vi "sub_panel_queue.vi"() -> ()   [LabVIEW 2024]
panel:
  out "Boolean":bool
  in  "knob":dbl(knob) scale=0.0..10.0
  out "numeric_test":dbl
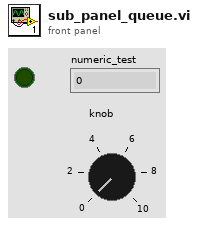
[diagram p1: front panel]
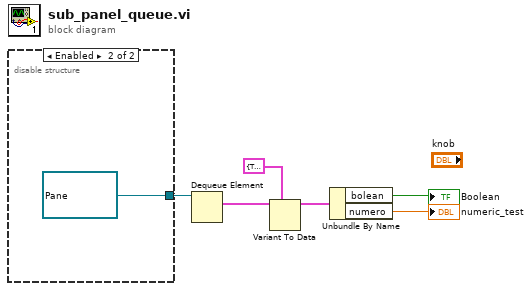
[diagram p0: block diagram]
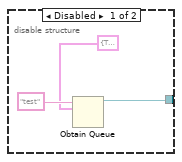
[diagram p2: hidden frame]
diagram:
  n1 = disable-structure shown="Enabled" {
    disable-tunnel: [w7 refnum<queue> refnum ("queue out")] -> w6
    frame Disabled {
      n2 = Obtain Queue(name (unnamed)="test", element data type=cluster{"bolean":bool, "numero":dbl} {"bolean"=TRUE, "numero"=0.0}) -> (queue out=w7:refnum<queue>)  [unwired: 3 in, 2 out]
    }
    frame Enabled {
    }
  }
  n3 = Dequeue Element(queue=w6) -> (element=w5:cluster{bool, dbl})  [unwired: 2 in, 3 out]
  n4 = Variant To Data(type=cluster{"bolean":bool, "numero":dbl} {"bolean"=TRUE, "numero"=0.0}, Variant=w5) -> (data=w3:cluster{"bolean":bool, "numero":dbl})  [unwired: 1 in, 1 out]
  n5 = Unbundle By Name(w3) -> ("bolean"=→"Boolean":bool, "numero"=→"numeric_test":dbl)
